vi "Get Channels.vi"(8 "error in (no error)":errorcluster, 11 "Transfer Configuration in":refnum<class "Transfer Configuration.lvclass">) -> (0 "error out":errorcluster, 2 "channels":T1[](array[typedef]) {"configuration"."string offset" format="%d bytes"}, 3 "Transfer Configuration out":refnum<class "Transfer Configuration.lvclass">)   [LabVIEW 2021, in "DSF Core.lvlib" / "Transfer Configuration.lvclass"]
uses:
  Transfer Configuration.lvclass
  Channel Configuration.ctl
  Typedefs/Core Channel Configuration.ctl
  Typedefs/DSF Data Type.ctl
  Typedefs/DSF Settings Info.ctl
  Transfer Configuration.lvclass/Transfer Configuration.ctl
  DSF Core.lvlib
  Channel/Channel Configuration.lvclass
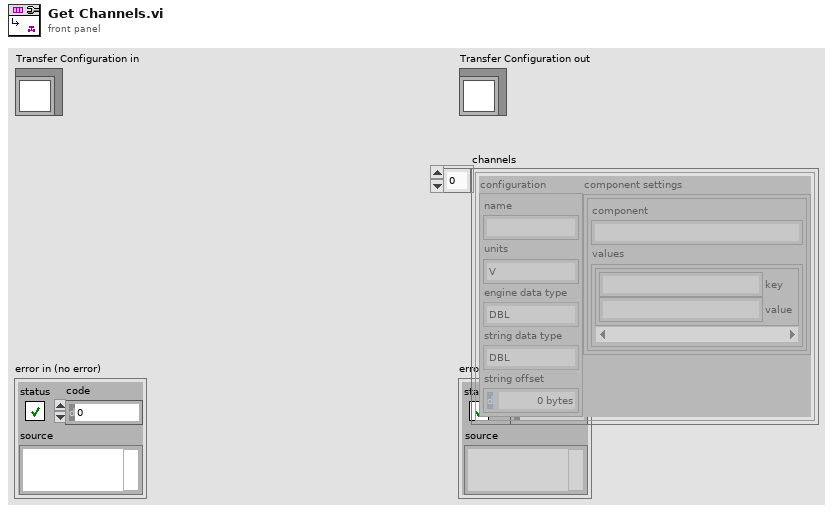
[diagram p1: front panel]
types:
  T1 = typedef "DSF Core.lvlib/Transfer Configuration.lvclass/Channel Configuration.ctl" = cluster{"configuration":T2, "component settings":T4[]}
  T2 = typedef "DSF Core.lvlib/Channel Configuration.lvclass/Core Channel Configuration.ctl" = cluster{"name":string, "units":string, "engine data type":T3, "string data type":T3, "string offset":u64}
  T3 = typedef "DSF Core.lvlib/DSF Data Type.ctl" = enum8{"Bool", "SGL", "DBL", "I8", "I16", "I32", "I64", "U8", "U16", "U32", "U64"}
  T4 = typedef "DSF Core.lvlib/DSF Settings Info.ctl" = cluster{"component":string, "values":cluster{"key":string, "value":string}[]}
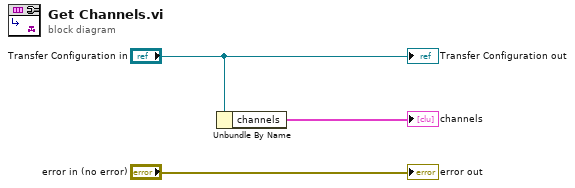
[diagram p0: block diagram]
diagram:
  n1 = Unbundle By Name("Transfer Configuration in") -> ("channels"=→"channels":T1[])
  "error out" <- "error in (no error)"
  "Transfer Configuration out" <- "Transfer Configuration in"
